vi "NewMenu.vi"(8 "error in":errorcluster, 10 "menu ref in":refnum<k9>, 11 "CEF_Repository in":refnum<class "CEF_Repository.lvclass">) -> (0 "error out":errorcluster, 2 "menu ref out":refnum<k9>, 3 "CEF_Repository out":refnum<class "CEF_Repository.lvclass">)   [LabVIEW 2025, in "CEF.lvlib" / "CEF_Repository.lvclass"]
doc: "Copyright 2017 National Instruments Corporation\n\nLicensed under the Apache License, Version 2.0 (the \"License\"); you may not use this file except in compliance with the License. You may obtain a copy of the License at http://www.apache.org/licenses/LICENSE-2.0\nUnless required by applicable law or agreed to in writing, software distributed under the License is distributed on an \"AS IS\" BASIS, WITHOUT WARRANTIES OR CONDITIONS OF ANY KIND, either express or implied. See the License for the specific language governing permissions and limitations under the License."
uses:
  CEF_Repository.lvclass
  <vilib>/Utility/miscctls.llb/LVMenuShortCut.ctl
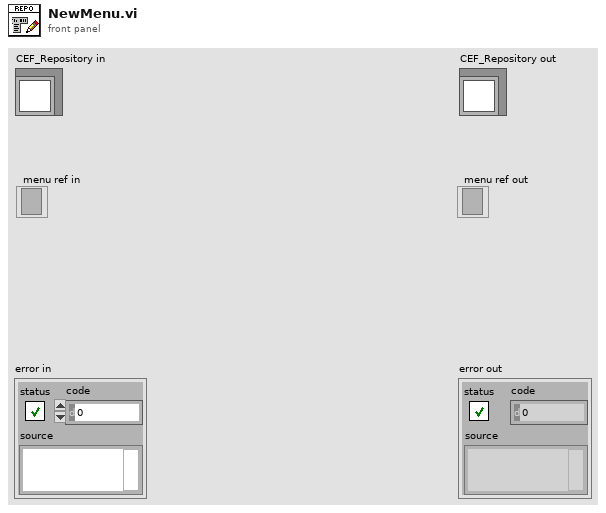
[diagram p1: front panel]
types:
  T1 = typedef "LVMenuShortCut.ctl" = cluster{"Include Shift Key?":bool, "Include Ctrl Key?":bool, "Shortcut Key":string}
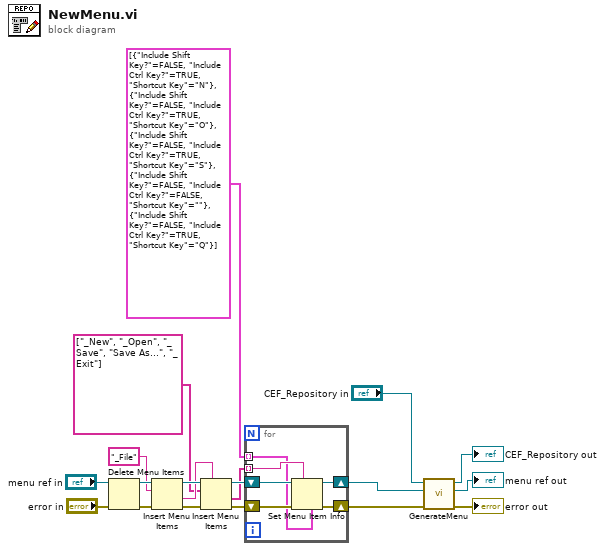
[diagram p0: block diagram]
diagram:
  n1 = Delete Menu Items(6:"error in", 9:"menu ref in") -> (0:w15:errorcluster, 3:w19:refnum<k9>)  [unwired: 2 in]
  n2 = Insert Menu Items(6:w15, 8:"_File", 9:w19) -> (0:w14:errorcluster, 1:w16:string, 3:w17:refnum<k9>)  [unwired: 3 in]
  n3 = Insert Menu Items(5:w16, 6:w14, 8:string[] ["_New", "_Open", "_Save", "Save As...", "_Exit"] ("item names"), 9:w17) -> (0:w11:errorcluster, 1:w10:string[], 3:w12:refnum<k9>)  [unwired: 2 in]
  n4 = for {
    shift-right: [w23] -> w2
    shift-left: w12 -> [w25]
    tunnel: w10 -> [w22] mode=indexing
    tunnel: T1[] [{"Include Shift Key?"=FALSE, "Include Ctrl Key?"=TRUE, "Shortcut Key"="N"}, {"Include Shift Key?"=FALSE, "Include Ctrl Key?"=TRUE, "Shortcut Key"="O"}, {"Include Shift Key?"=FALSE, "Include Ctrl Key?"=TRUE, "Shortcut Key"="S"}, {"Include Shift Key?"=FALSE, "Include Ctrl Key?"=FALSE, "Shortcut Key"=""}, {"Include Shift Key?"=FALSE, "Include Ctrl Key?"=TRUE, "Shortcut Key"="Q"}] -> [w20] mode=indexing
    shift-right: [w21] -> w1
    shift-left: w11 -> [w24]
    n5 = Set Menu Item Info(4:w20, 7:w22, 8:w24, 11:w25) -> (0:w21:errorcluster, 3:w23:refnum<k9>)  [unwired: 3 in]
  }
  n6 = call-dynamic "GenerateMenu.vi"("error in"=w1, "menu ref in"=w2, "CEF_Repository in"="CEF_Repository in") -> ("error out"=→"error out":errorcluster, "menu ref out"=→"menu ref out":refnum<k9>, "CEF_Repository out"=→"CEF_Repository out":refnum<class "CEF_Repository.lvclass">)  [unwired: 6 in]
